vi "Launch Live Report Viewer.vi"(8 "error in":errorcluster, 11 "Report in":refnum<class "Report.lvclass">) -> (0 "error out":errorcluster, 3 "Report out":refnum<class "Report.lvclass">)   [LabVIEW 2023, in "Report.lvlib" / "Report.lvclass"]
doc: "This is a wrapper function to provide asynchronous VI lauching of the live report viewer. \n\nAsynchronous launching is critical because it allows data capture/creation and update to continue in the background while the user is analyzing the data in real time. \n\nTo launch asynchronously a strictly typed vi reference must be passed into the call asnychronously application tool. That cannot be done with the dynamically dispatched Read Live Report VI. However, a static dispatched wrapper such as this can call the child function dynamically after it has been called. That is the purpose of this wrapper."
uses:
  Report.lvclass
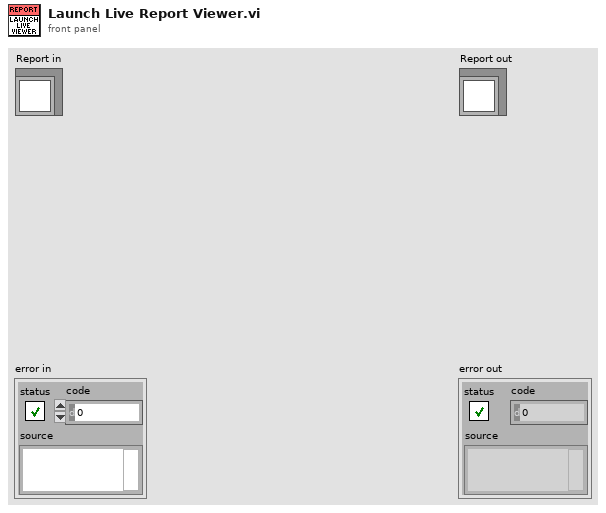
[diagram p1: front panel]
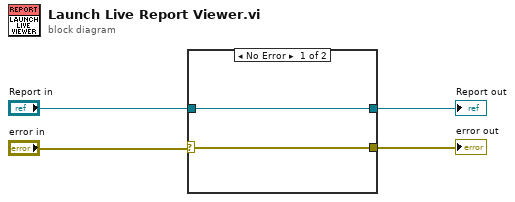
[diagram p0: block diagram]
diagram:
  n1 = case shown="No Error" "error in" {
    selector: "error in" -> [w5 w8]
    tunnel: [w5 w8] -> w4
    tunnel: [w6 w7] -> w2
    tunnel: "Report in" -> [w6 w7]
    frame No Error {
    }
    frame Error {
    }
  }
  "error out" <- w4
  "Report out" <- w2
